vi "Application Name.vi"(11 "Sequence Context In":refnum<k7>) -> (3 "Application:Name":string)   [LabVIEW 2020]
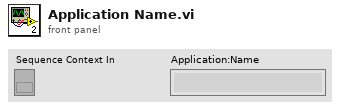
[diagram p1: front panel]
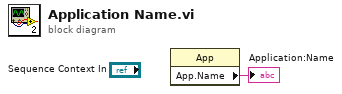
[diagram p0: block diagram]
diagram:
  n1 = property class="App"() -> ("App.Name"=→"Application:Name":string)  [unwired: 2 in, 2 out]
